vi "QuadRotor_Monitoring_LV4_NOMotorController.vi"() -> ()   [LabVIEW 2015]
uses:
  <vilib>/Instr/_visa.llb/VISA Set IO Buffer Mask.ctl
  <vilib>/Instr/_visa.llb/VISA Configure Serial Port (Instr).vi
panel:
  out "GPS_TRANSPORT_Distance":dbl(slide) scale=0.0..200.0
  out "GPS_Home_Distance":dbl(slide) scale=0.0..200.0
  out "GPS_Speed_Gaud":ext(knob) scale=0.0..100.0
  out "GPS_LON_TRANSPORT":ext format="%#.7f"
  out "GPS_LAT_TRANSPORT":ext format="%#.7f"
  out "GPS_LON_HOME":ext format="%#.7f"
  out "GPS_LAT_HOME":ext format="%#.7f"
  in  "LON_TRANSPORT":i32=1001113510
  in  "LAT_TRANSPORT":i32=200300620
  in  "LON_HOME":i32=1001110710
  in  "LAT_HOME":i32=200292880
  out "(GPS_numSat)":u16(slide) scale=0.0..20.0 scale format="%#_4g"
  out "return count 2":u32
  out "Roob":i32
  out "Altitude_(Auto)":ext format="%#_3g"
  in  "Set_ATL_(Auto)":dbl=12.0
  out "string":string
  out "Mode":ext format="%.2f"
  out "Altitude":dbl(slide) scale=0.0..20.0
  out "Altitude":ext format="%.2f"
  out "Yaw":dbl(knob) scale=-180.0..180.0
  out "Pitch":dbl(knob) scale=-90.0..90.0
  out "Roll":dbl(knob) scale=-90.0..90.0
  in  "Write to Quad":bool
  out "Header_58":u8
  out "GPS_LONGTITUDE":ext format="%#.7f"
  out "GPS_LATTITUDE":ext format="%#.7f"
  out "return count":u32
  in  "stop":bool
  in  "VISA Serial Data":refnum<visa-resource-name>
  # "Quad Rotor Monitoring and Control with GPS Waypoint"
  # "Quad Rotor System monitoring and controller"
  # "Ex  13.8591411 = 138591411 , 100.5231704 = 1005231704 Using in integer  I32"
  # "GPS Status and Monitoring"
  # "Km/h"
  # "GPS Position Write to Quad"
  # "9 Point"
  # "10 Point"
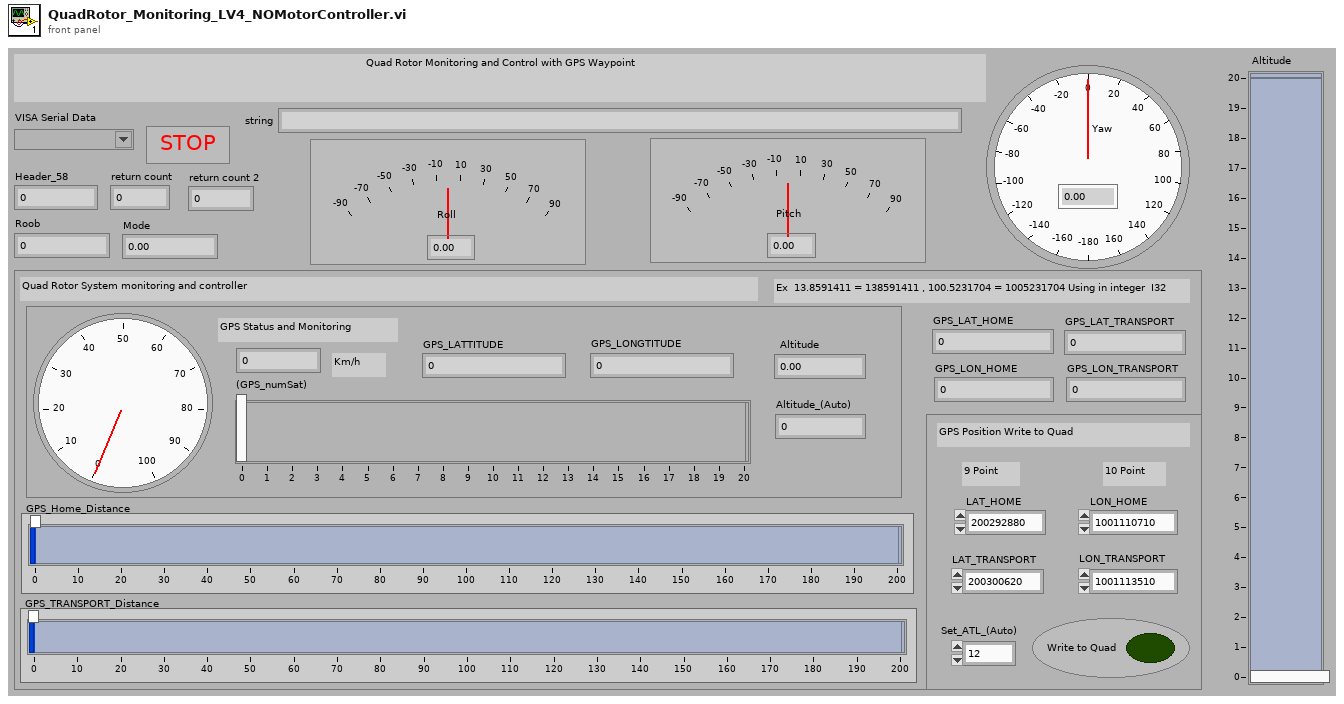
[diagram p1: front panel]
types:
  T1 = typedef "VISA Set IO Buffer Mask.ctl" = u16
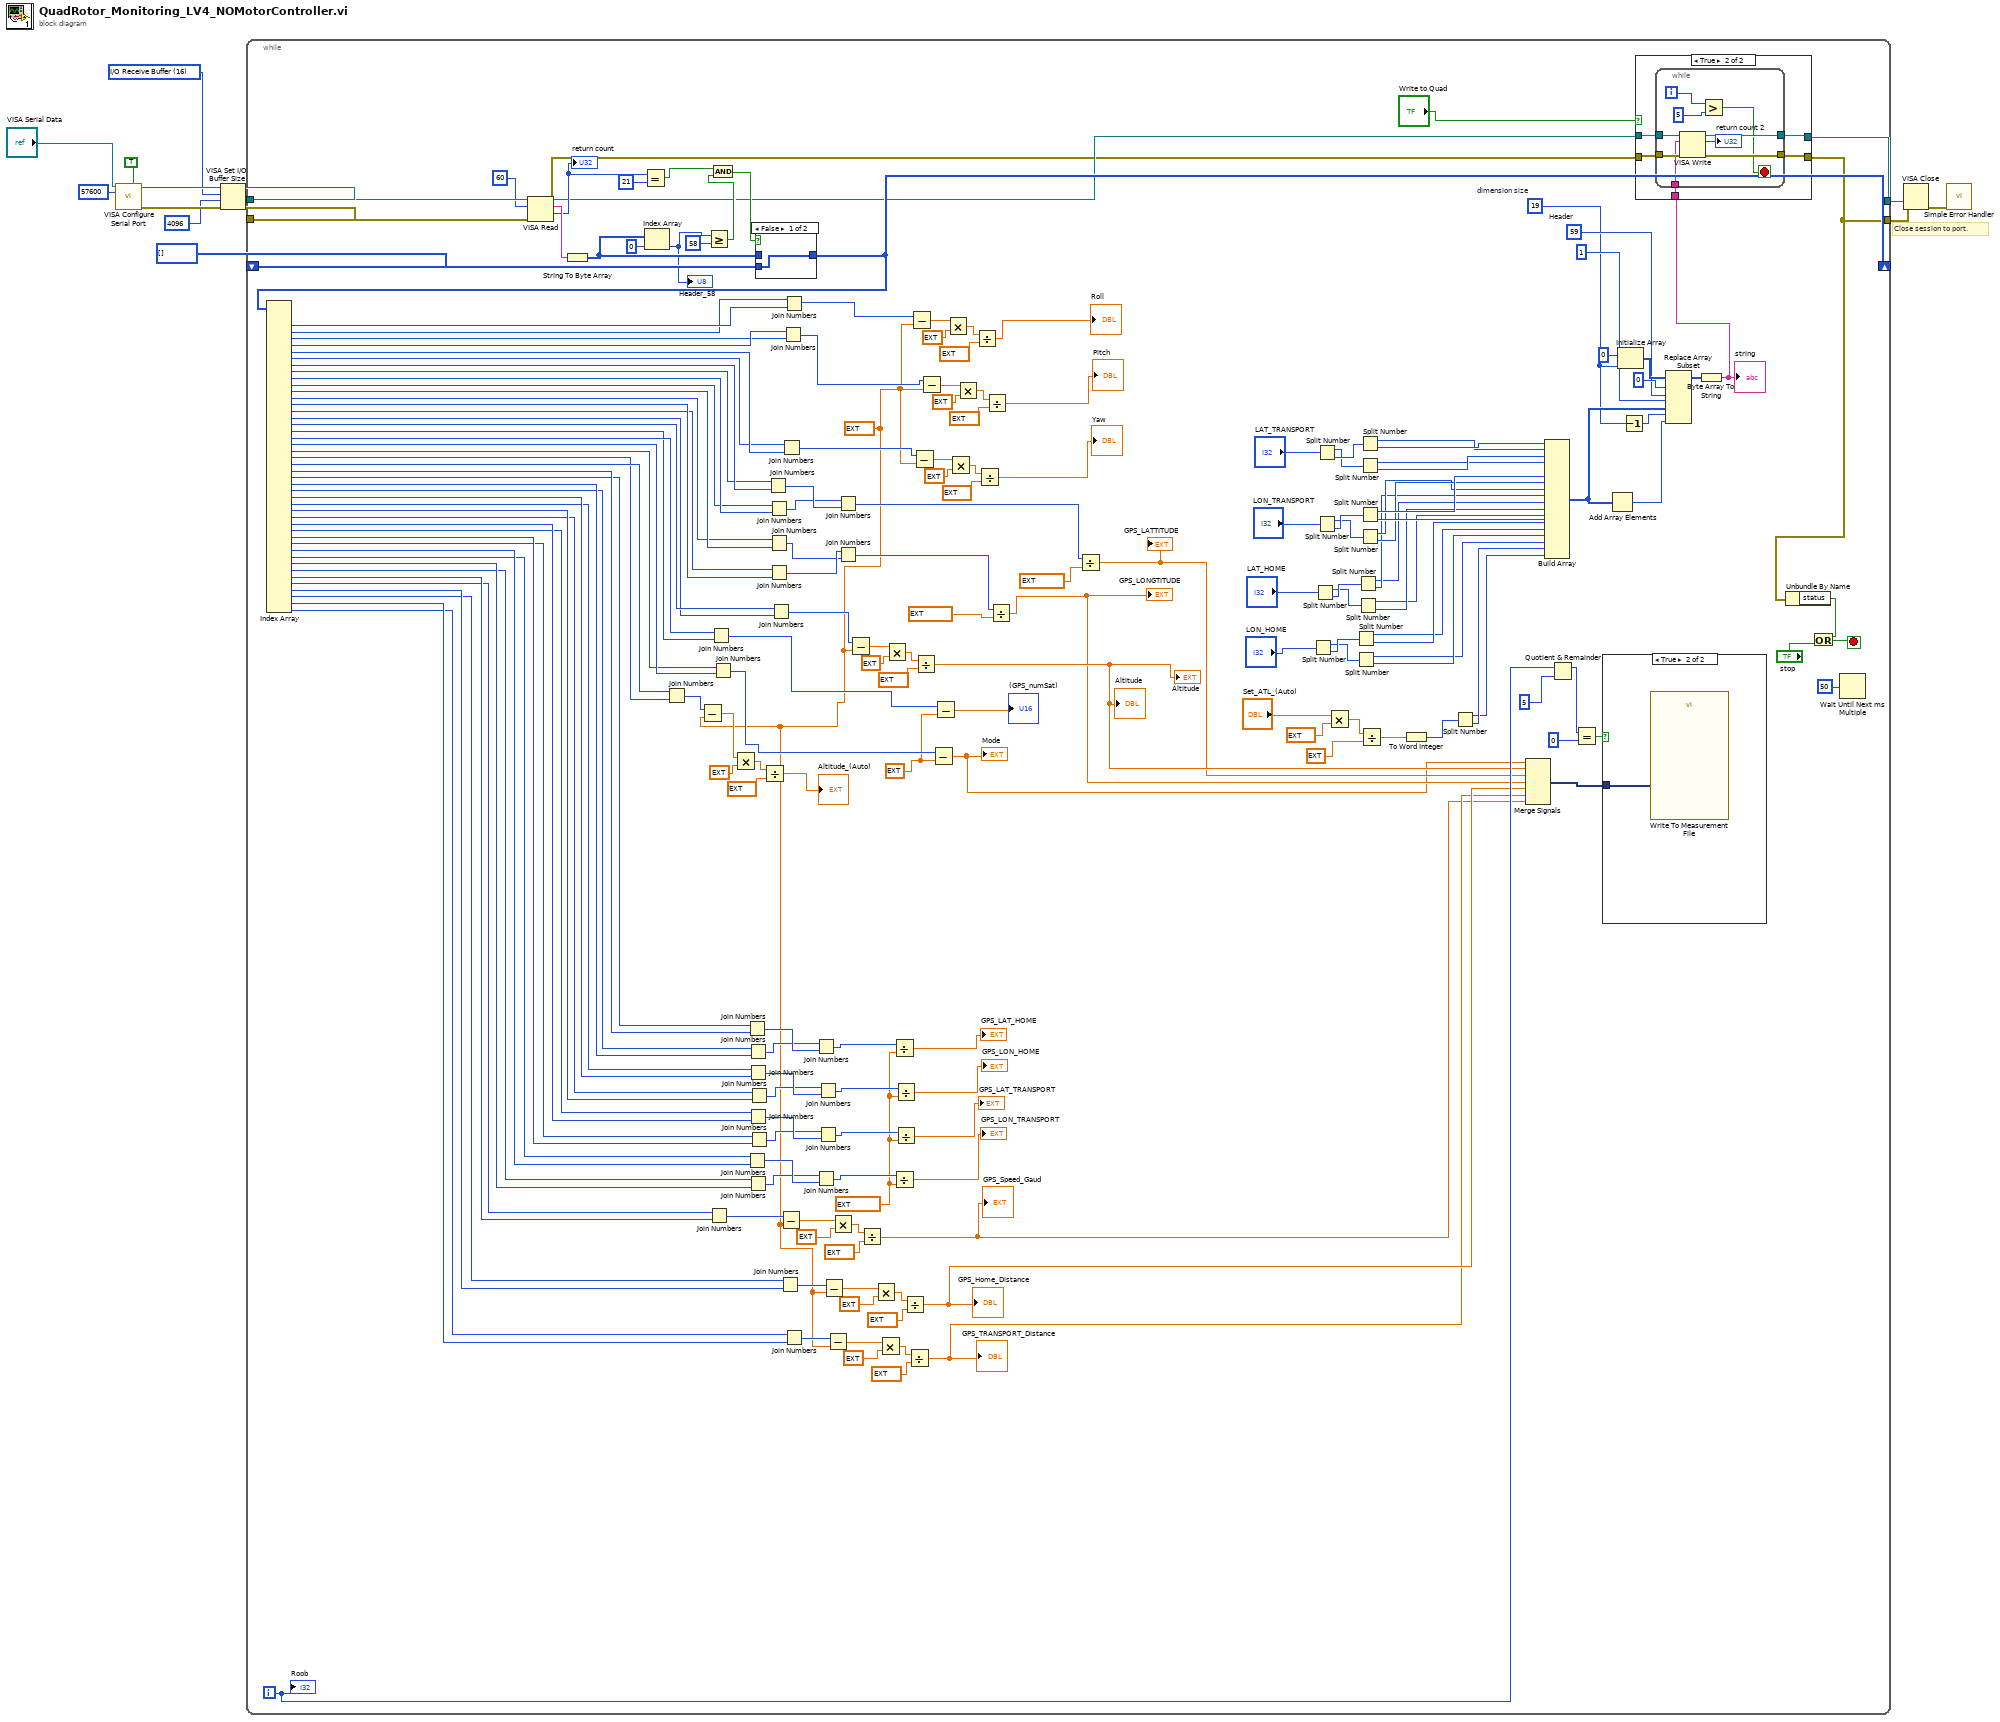
[diagram p0: block diagram]
diagram:
  w10 = T1 16 items=["I/O Receive Buffer"=16, "I/O Transmit Buffer"=32, "I/O Receive and Transmit Buffer"=48] ("Mask")
  # "Close session to port."
  n1 = call-poly "VISA Configure Serial Port"("VISA resource name"="VISA Serial Data", "Enable Termination\nChar (T)"=TRUE ("Enable Termination\nChar (T)"), "baud rate (9600)"=u32 57600) -> ("VISA resource name out"=w12:refnum<visa-resource-name>, "error out"=w11:errorcluster)  [unwired: 7 in, 4 out]
  n2 = VISA Set I/O Buffer Size(VISA resource name=w12, mask (16)=w10, size (4096)=u32 4096, error in (no error)=w11) -> (VISA resource name out=w8:refnum<visa-resource-name>, error out=w6:errorcluster)
  n3 = while {
    tunnel: [w171] -> w7
    tunnel: w8 -> [w212]
    tunnel: [w170] -> w5
    tunnel: w6 -> [w211]
    shift-right: [w181] -> _
    shift-left: u8[] [] ("unsigned byte array") -> [w182]
    i -> [w81]
    stop <- w215 stop-if-true
    w59 = ext 10000000.0 ("y")
    w92 = 19  # dimension size
    w139 = u8 59  # Header
    w85 = ext 255.0 ("y")
    w36 = ext 32767.0 ("y")
    n4 = VISA Read(VISA resource name=w212, byte count=u32 60, error in (no error)=w211) -> (VISA resource name out=w173:refnum<visa-resource-name>, read buffer=w185:string, return count=w178:u32, error out=w172:errorcluster)
    "return count" <- w178
    n5 = String To Byte Array(string=w185) -> (unsigned byte array=w183:u8[])
    n6 = Equal?(x=w178, y=u32 21) -> (x = y?=w176:bool)
    n7 = Index Array(array=w183, index=0) -> (element=w175:u8)
    "Header_58" <- w175
    n8 = Greater Or Equal?(x=w175, y=u8 58) -> (x >= y?=w180:bool)
    n9 = And(x=w176, y=w180) -> (x .and. y?=w179:bool)
    n10 = case shown="False" w179 {
      tunnel: w183 -> [_ w234]
      tunnel: [w233 w234] -> w181
      tunnel: w182 -> [w233 _]
      frame False {
      }
      frame True {
      }
    }
    n11 = Index Array(array=w181) -> (element #2=w205:u8, element #3=w204:u8, element #4=w202:u8, element #5=w203:u8, element #6=w209:u8, element #7=w208:u8, element #8=w207:u8, element #9=w206:u8, element #10=w166:u8, element #11=w165:u8, element #12=w162:u8, element #13=w161:u8, element #14=w160:u8, element #15=w159:u8, element #16=w150:u8, element #17=w156:u8, element #18=w148:u8, element #19=w149:u8, element #20=w147:u8, element #21=w146:u8, element #22=w103:u8, element #23=w104:u8, element #24=w35:u8, element #25=w34:u8, element #26=w33:u8, element #27=w32:u8, element #28=w31:u8, element #29=w30:u8, element #30=w29:u8, element #31=w28:u8, element #32=w27:u8, element #33=w26:u8, element #34=w25:u8, element #35=w24:u8, element #36=w23:u8, element #37=w22:u8, element #38=w21:u8, element #39=w20:u8, element #40=w19:u8, element #41=w18:u8, element #42=w17:u8, element #43=w16:u8, element #44=w15:u8, element #45=w14:u8)  [unwired: 45 in, 1 out]
    n12 = Join Numbers(hi=w104, lo=w103) -> ((hi.lo)=w102:u16)
    n13 = Subtract(x=w102, y=w36) -> (x-y=w98:ext)
    n14 = Join Numbers(hi=w18, lo=w19) -> ((hi.lo)=w54:u16)
    n15 = Join Numbers(hi=w149, lo=w148) -> ((hi.lo)=w84:u16)
    n16 = Join Numbers(hi=w146, lo=w147) -> ((hi.lo)=w87:u16)
    n17 = Multiply(x=w98, y=ext 100.0) -> (x*y=w100:ext)
    n18 = Join Numbers(hi=w34, lo=w35) -> ((hi.lo)=w75:u16)
    n19 = Join Numbers(hi=w22, lo=w23) -> ((hi.lo)=w66:u16)
    n20 = Join Numbers(hi=w32, lo=w33) -> ((hi.lo)=w74:u16)
    n21 = Join Numbers(hi=w20, lo=w21) -> ((hi.lo)=w65:u16)
    n22 = Join Numbers(hi=w30, lo=w31) -> ((hi.lo)=w72:u16)
    n23 = Join Numbers(hi=w26, lo=w27) -> ((hi.lo)=w69:u16)
    n24 = Join Numbers(hi=w28, lo=w29) -> ((hi.lo)=w71:u16)
    n25 = Join Numbers(hi=w24, lo=w25) -> ((hi.lo)=w68:u16)
    n26 = Divide(x=w100, y=ext 32767.0) -> (x/y=→"Altitude_(Auto)":ext)
    n27 = Join Numbers(hi=w206, lo=w207) -> ((hi.lo)=w164:u16)
    n28 = Join Numbers(hi=w165, lo=w166) -> ((hi.lo)=w163:u16)
    n29 = Join Numbers(hi=w161, lo=w162) -> ((hi.lo)=w144:u16)
    n30 = Join Numbers(hi=w159, lo=w160) -> ((hi.lo)=w145:u16)
    n31 = Join Numbers(hi=w156, lo=w150) -> ((hi.lo)=w151:u16)
    n32 = Join Numbers(hi=w16, lo=w17) -> ((hi.lo)=w49:u16)
    n33 = Subtract(x=w54, y=w36) -> (x-y=w57:ext)
    n34 = Join Numbers(hi=w208, lo=w209) -> ((hi.lo)=w191:u16)
    n35 = Join Numbers(hi=w203, lo=w202) -> ((hi.lo)=w186:u16)
    n36 = Join Numbers(hi=w204, lo=w205) -> ((hi.lo)=w200:u16)
    n37 = Join Numbers(hi=w14, lo=w15) -> ((hi.lo)=w44:u16)
    n38 = Join Numbers(hi=w74, lo=w75) -> ((hi.lo)=w73:u32)
    n39 = Join Numbers(hi=w65, lo=w66) -> ((hi.lo)=w64:u32)
    n40 = Join Numbers(hi=w71, lo=w72) -> ((hi.lo)=w70:u32)
    n41 = Join Numbers(hi=w68, lo=w69) -> ((hi.lo)=w67:u32)
    n42 = Subtract(x=w49, y=w36) -> (x-y=w52:ext)
    n43 = Subtract(x=w44, y=w36) -> (x-y=w47:ext)
    n44 = Multiply(x=w57, y=ext 100.0) -> (x*y=w58:ext)
    n45 = Join Numbers(hi=w163, lo=w164) -> ((hi.lo)=w168:u32)
    n46 = Join Numbers(hi=w145, lo=w144) -> ((hi.lo)=w158:u32)
    n47 = Subtract(x=w151, y=w36) -> (x-y=w155:ext)
    n48 = Divide(x=w58, y=ext 32767.0) -> (x/y=w38:ext)
    "GPS_Speed_Gaud" <- w38
    n49 = Multiply(x=w52, y=ext 200.0) -> (x*y=w53:ext)
    n50 = Multiply(x=w47, y=ext 200.0) -> (x*y=w48:ext)
    n51 = Multiply(x=w155, y=ext 100.0) -> (x*y=w153:ext)
    n52 = Divide(x=w73, y=w59) -> (x/y=→"GPS_LAT_HOME":ext)
    n53 = Divide(x=w64, y=w59) -> (x/y=→"GPS_LON_TRANSPORT":ext)
    n54 = Divide(x=w70, y=w59) -> (x/y=→"GPS_LON_HOME":ext)
    n55 = Divide(x=w67, y=w59) -> (x/y=→"GPS_LAT_TRANSPORT":ext)
    n56 = Divide(x=w53, y=ext 32767.0) -> (x/y=w40:ext)
    "GPS_Home_Distance" <- w40
    n57 = Divide(x=w48, y=ext 32767.0) -> (x/y=w39:ext)
    "GPS_TRANSPORT_Distance" <- w39
    n58 = Subtract(x=w200, y=w36) -> (x-y=w199:ext)
    n59 = Subtract(x=w191, y=w36) -> (x-y=w195:ext)
    n60 = Divide(x=w153, y=ext 32767.0) -> (x/y=w43:ext)
    "Altitude" <- w43
    "Altitude" <- w43
    n61 = Subtract(x=w186, y=w36) -> (x-y=w190:ext)
    n62 = Subtract(x=w87, y=w85) -> (x-y=w37:ext)
    "Mode" <- w37
    n63 = Subtract(x=w84, y=w85) -> (x-y=→"(GPS_numSat)":ext)
    n64 = Multiply(x=w199, y=ext 180.0) -> (x*y=w197:ext)
    n65 = Multiply(x=w195, y=ext 180.0) -> (x*y=w193:ext)
    n66 = Multiply(x=w190, y=ext 180.0) -> (x*y=w188:ext)
    n67 = Divide(x=w197, y=ext 32767.0) -> (x/y=→"Roll":ext)
    n68 = Divide(x=w193, y=ext 32767.0) -> (x/y=→"Yaw":ext)
    n69 = Divide(x=w188, y=ext 32767.0) -> (x/y=→"Pitch":ext)
    n70 = Divide(x=w158, y=ext 10000000.0) -> (x/y=w41:ext)
    "GPS_LONGTITUDE" <- w41
    n71 = Divide(x=w168, y=ext 10000000.0) -> (x/y=w42:ext)
    "GPS_LATTITUDE" <- w42
    n72 = Split Number(x="LON_HOME") -> (hi(x)=w132:u16, lo(x)=w133:u16)
    n73 = Split Number(x="LAT_HOME") -> (hi(x)=w134:u16, lo(x)=w135:u16)
    n74 = Split Number(x="LON_TRANSPORT") -> (hi(x)=w136:u16, lo(x)=w137:u16)
    n75 = Split Number(x="LAT_TRANSPORT") -> (hi(x)=w114:u16, lo(x)=w115:u16)
    n76 = Multiply(x="Set_ATL_(Auto)", y=ext 32767.0) -> (x*y=w107:ext)
    n77 = Split Number(x=w133) -> (hi(x)=w118:u8, lo(x)=w119:u8)
    n78 = Split Number(x=w132) -> (hi(x)=w116:u8, lo(x)=w117:u8)
    n79 = Split Number(x=w135) -> (hi(x)=w122:u8, lo(x)=w123:u8)
    n80 = Split Number(x=w134) -> (hi(x)=w120:u8, lo(x)=w121:u8)
    n81 = Split Number(x=w137) -> (hi(x)=w126:u8, lo(x)=w127:u8)
    n82 = Split Number(x=w136) -> (hi(x)=w124:u8, lo(x)=w125:u8)
    n83 = Split Number(x=w115) -> (hi(x)=w130:u8, lo(x)=w131:u8)
    n84 = Split Number(x=w114) -> (hi(x)=w128:u8, lo(x)=w129:u8)
    n85 = Divide(x=w107, y=ext 100.0) -> (x/y=w105:ext)
    n86 = To Word Integer(number=w105) -> (16bit integer=w108:i16)
    n87 = Split Number(x=w108) -> (hi(x)=w109:u8, lo(x)=w110:u8)
    n88 = Merge Signals(w37, w43, w42, w41, w40, w39, w38) -> (w83:dynamicdata)
    n89 = Build Array(w131, w130, w129, w128, w127, w126, w125, w124, w123, w122, w121, w120, w119, w118, w117, w116, w110, w109) -> (w95:u8[])
    n90 = Quotient & Remainder(x=w81, y=u32 5) -> (x-y*floor(x/y)=w78:u32)  [unwired: 1 out]
    n91 = Equal?(x=w78, y=u32 0) -> (x = y?=w80:bool)
    n92 = case shown="True" w80 {
      tunnel: w83 -> [_ w216]
      frame False {
      }
      frame True {
        n93 = call "Write To Measurement File"("Signals"=w216) -> ()  [unwired: 16 in, 3 out]
      }
    }
    n94 = Add Array Elements(numeric array=w95) -> (sum=w94:u8)
    n95 = Initialize Array(u8 0, w92) -> (w143:u8[])
    n96 = Decrement(x=w92) -> (x-1=w93:i32)
    n97 = Replace Array Subset(array=w143, new element #1=w139, index #1=0 ("index"), new element #2=w95, index #2=1 ("index"), new element #3=w94, index #3=w93) -> (w138:u8[])
    n98 = Byte Array To String(unsigned byte array=w138) -> (string=w113:string)
    "string" <- w113
    n99 = case shown="True" "Write to Quad" {
      tunnel: w173 -> [w217 w223]
      tunnel: w172 -> [w218 w220]
      tunnel: [w217 w222] -> w171
      tunnel: [w218 w221] -> w170
      tunnel: w113 -> [_ w219]
      frame False {
      }
      frame True {
        n100 = while {
          tunnel: w223 -> [w232]
          tunnel: [w231] -> w222
          tunnel: [w230] -> w221
          tunnel: w220 -> [w229]
          tunnel: w219 -> [w228]
          i -> [w226]
          stop <- w224 stop-if-true
          n101 = VISA Write(VISA resource name=w232, write buffer=w228, error in (no error)=w229) -> (VISA resource name out=w231:refnum<visa-resource-name>, return count=→"return count 2":u32, error out=w230:errorcluster)
          n102 = Greater?(x=w226, y=5) -> (0:w224:bool)
        }
      }
    }
    n103 = Unbundle By Name(w170) -> ("status"=w213:bool)
    n104 = Or(x=w213, y="stop") -> (x .or. y?=w215:bool)
    n105 = Wait Until Next ms Multiple(millisecond multiple=u32 50) -> ()  [unwired: 1 out]
    "Roob" <- w81
  }
  n106 = VISA Close(VISA resource name=w7, error in (no error)=w5) -> (error out=w9:errorcluster)
  n107 = call <vilib>:"Simple Error Handler.vi"("error in (no error)"=w9) -> ()  [unwired: 1 in, 8 out]
